vi "QControl_Graph_Example.vi"() -> ()   [LabVIEW 2017]
uses:
  QControl_Graph/QControl_Graph.lvclass
  <vilib>/ptbypt/NI_PtbyPt.lvlib
panel:
  out "Status":string
  out "XY Graph":cluster{dbl[], dbl[]}[](graph)
  # "Position the mouse over the graph, and use the scroll wheel to zoom in and out.  \n1. No modifiers, just straight scroll wheel.  This zooms on the X-Axis to zoom in and out\n2. SHIFT, changes the zoom to be on the Y-Axis\n3. CTRL, changes to a pan mode, sliding on the X-Axis with the scroll wheel\n4. CTRL SHIFT, pans on the Y-Axis with the scroll wheel"
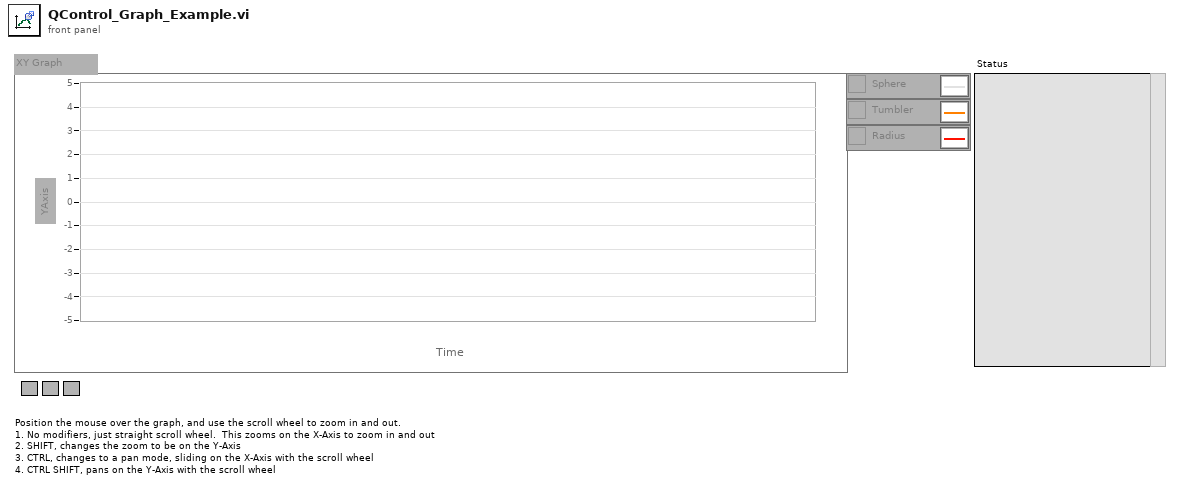
[diagram p1: front panel]
types:
  T1 = typedef "QControl_Graph.lvclass/Actions.ctl" = enum16{"Undefined", "BGK Color", "Highlight Plot", "Mouse Zoom", "Show Cursors", "Cursor Properties", "Show Markers"}
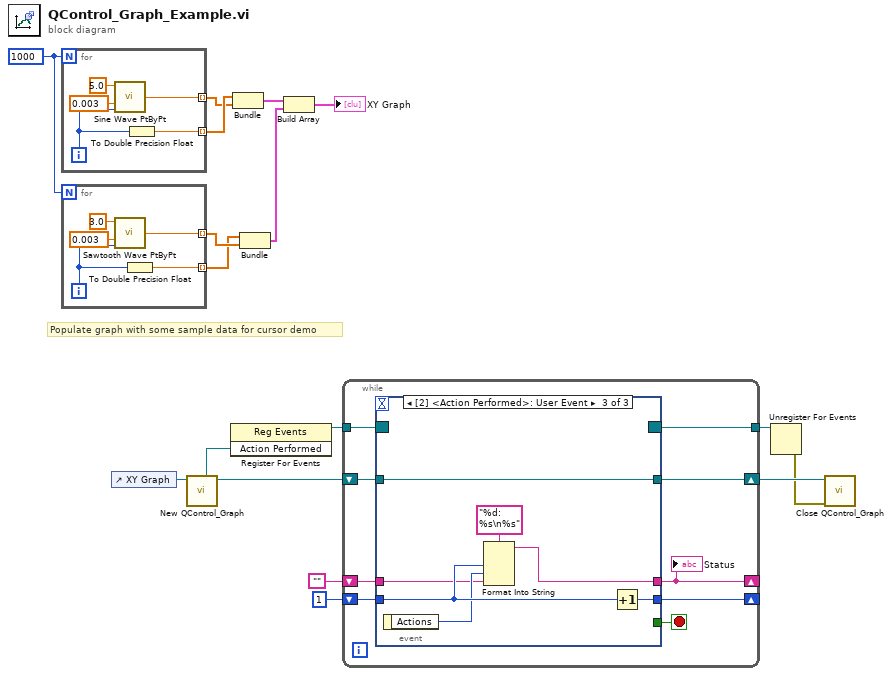
[diagram p0: block diagram]
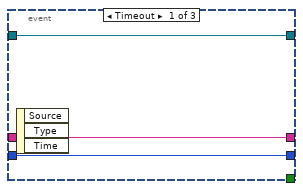
[diagram p2: hidden frame]
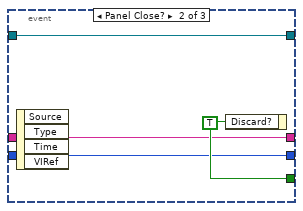
[diagram p3: hidden frame]
diagram:
  w2 = 1000
  # "Populate graph with some sample data for cursor demo"
  n1 = for {
    N: w2 -> [_]
    tunnel: [w22] -> w7 mode=indexing
    tunnel: [w18] -> w8 mode=indexing
    i -> [w21]
    n2 = call <vilib>:"Sine Wave PtByPt.vi"("time"=w21, "frequency"=0.003, "amplitude"=5.0) -> ("sine wave"=w22:dbl)  [unwired: 1 in]
    n3 = To Double Precision Float(number=w21) -> (double precision float=w18:dbl)
  }
  n4 = for {
    N: w2 -> [_]
    tunnel: [w27] -> w5 mode=indexing
    tunnel: [w23] -> w4 mode=indexing
    i -> [w26]
    n5 = call <vilib>:"Sawtooth Wave PtByPt.vi"("time"=w26, "frequency"=0.003, "amplitude"=3.0) -> ("sawtooth wave"=w27:dbl)  [unwired: 1 in]
    n6 = To Double Precision Float(number=w26) -> (double precision float=w23:dbl)
  }
  n7 = control-ref of="XY Graph"() -> (w17:refnum<vi>)
  n8 = call "New QControl_Graph.vi"("Reference"=w17) -> ("QControl_Graph out"=w16:refnum<class "QControl_Graph.lvclass">, "Action Performed"=w13:refnum<user-event>)  [unwired: 8 in, 1 out]
  n9 = register-events(w13) -> (reference out=w14:refnum<event-registration>)  [unwired: 2 in, 1 out]
  n10 = Bundle(w8, w7) -> (w6:cluster{dbl[], dbl[]})  [unwired: 1 in]
  n11 = Bundle(w4, w5) -> (w3:cluster{dbl[], dbl[]})  [unwired: 1 in]
  n12 = Build Array(w6, w3) -> (→"XY Graph":cluster{dbl[], dbl[]}[])
  n13 = while {
    shift-right: [w35] -> w15
    shift-left: w16 -> [w36]
    tunnel: w14 -> [w33]
    tunnel: [w32] -> w12
    shift-right: [w28] -> _
    shift-left: "" -> [w31]
    shift-right: [w29] -> _
    shift-left: 1 -> [w30]
    stop <- w34 stop-if-true
    n14 = event shown="[2] <Action Performed>: User Event" {
      selector: w33 -> [_ _ _]
      dyn-events: [_ _ _] -> w32
      timeout: _ -> [_ _ _]
      tunnel: w36 -> [w39 w43 w50]
      tunnel: [w39 w43 w50] -> w35
      tunnel: [_ w42 _] -> w34
      tunnel: w31 -> [w38 w41 w44]
      tunnel: [w38 w41 w49] -> w28
      tunnel: w30 -> [w37 w40 w46]
      tunnel: [w37 w40 w48] -> w29
      event Timeout {
        n15 = event-data() -> ()  [unwired: 1 in, 3 out]
      }
      event Panel Close? {
        w42 = TRUE ("Discard?")
        n16 = event-data() -> ()  [unwired: 1 in, 4 out]
        n17 = event-data("Discard?"=w42) -> ()  [unwired: 1 in, 1 out]
      }
      event User Event {
        n18 = event-data() -> ("Actions"=w45:T1)  [unwired: 1 in]
        n19 = Format Into String(format string="%d: %s\n%s", w46, w45, w44) -> (resulting string=w49:string)  [unwired: 2 in, 1 out]
        n20 = Increment(x=w46) -> (x+1=w48:i32)
      }
    }
    "Status" <- w28
  }
  n21 = Unregister For Events(event registration refnum=w12) -> (error out=w11:errorcluster)  [unwired: 1 in]
  n22 = call "Close QControl_Graph.vi"("error in (no error)"=w11, "QControl_Graph in"=w15) -> ()  [unwired: 9 in, 1 out]
